vi "LinearKFLOP.vi"(8 "Array":dbl[](array[numeric]), 10 "error in (no error)":errorcluster, 11 "new reference":refnum<k24>) -> (2 "error out":errorcluster, 3 "new reference 2":refnum<k24>)   [LabVIEW 2017]
uses:
  C:/KMotion434/KMotion/Release/KMotion_dotNet.dll
panel:
  in  "y":bool
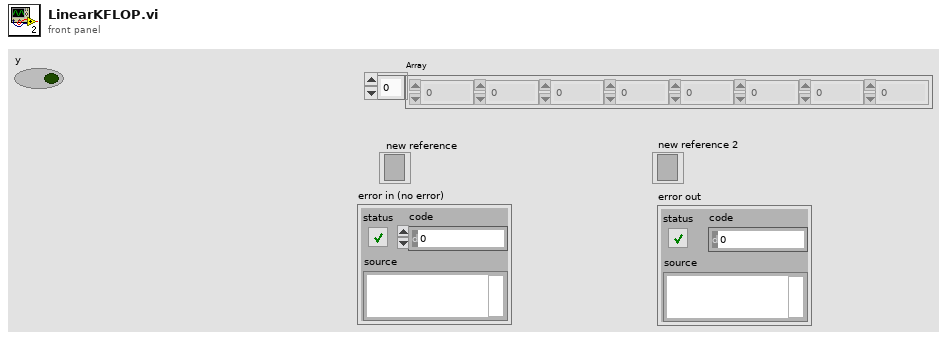
[diagram p1: front panel]
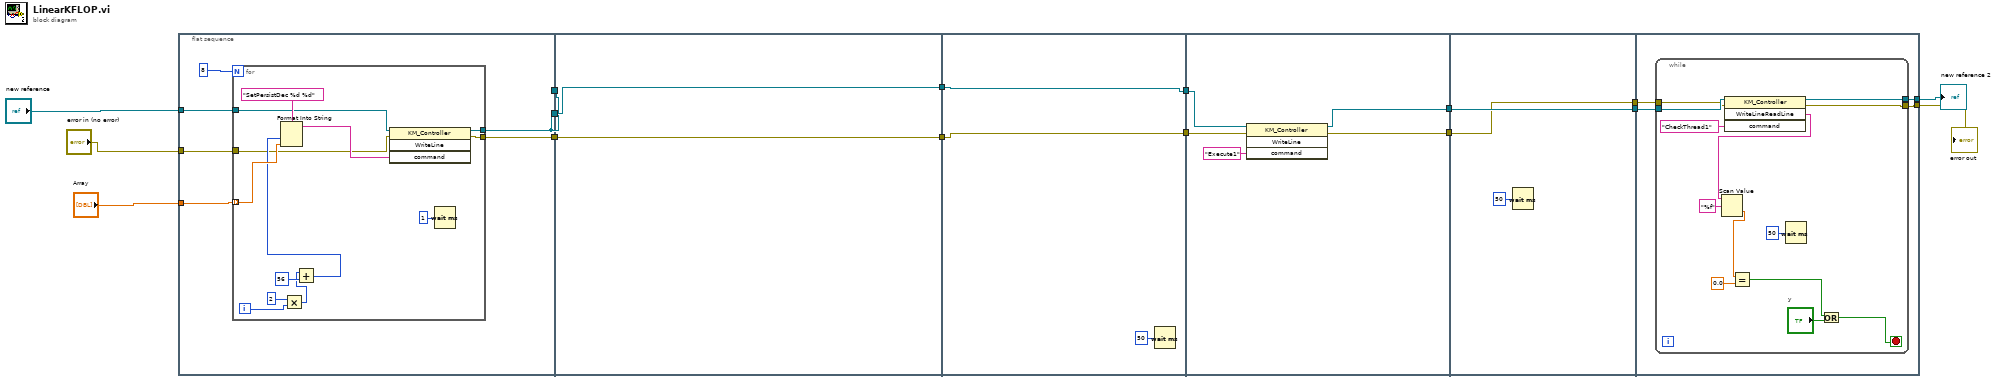
[diagram p0: block diagram]
diagram:
  n1 = flat-sequence {
    tunnel: "new reference" -> [w21]
    tunnel: "Array" -> [w20]
    tunnel: [w19] -> w15
    tunnel: [w19] -> w14
    tunnel: "error in (no error)" -> [w18]
    tunnel: [w17] -> w7
    tunnel: w15 -> [_]
    tunnel: w14 -> [w37]
    tunnel: [w37] -> w13
    tunnel: [w36] -> w8
    tunnel: w7 -> [w36]
    tunnel: [w39] -> w16
    tunnel: w13 -> [w39]
    tunnel: w8 -> [w38]
    tunnel: [w38] -> w6
    tunnel: w16 -> [w45]
    tunnel: [w44] -> w12
    tunnel: w6 -> [w41]
    tunnel: [w42] -> w4
    tunnel: w12 -> [w48]
    tunnel: [w48] -> w11
    tunnel: [w46] -> w5
    tunnel: w4 -> [w46]
    tunnel: w11 -> [w52]
    tunnel: w5 -> [w51]
    tunnel: [w50] -> w3
    tunnel: [w49] -> w2
    frame #0 {
      n2 = for {
        N: 8 -> [_]
        tunnel: w21 -> [w29]
        tunnel: w20 -> [w33] mode=indexing
        tunnel: [w32] -> w19
        tunnel: w18 -> [w24]
        tunnel: [w23] -> w17
        i -> [w27]
        n3 = Multiply(x=2, y=w27) -> (x*y=w26:i32)
        n4 = Add(x=w26, y=56) -> (x+y=w30:i32)
        n5 = Format Into String(format string="SetPersistDec %d %d" ("command"), w30, w33) -> (resulting string=w35:string)  [unwired: 2 in, 1 out]
        n6 = invoke class="KM_Controller" method="WriteLine"(reference=w29, error in=w24, "command"=w35) -> (reference out=w32:refnum<k24>, error out=w23:errorcluster)  [unwired: 1 in, 2 out]
        n7 = Wait (ms)(milliseconds to wait=u32 1) -> ()  [unwired: 1 out]
      }
    }
    frame #1 {
    }
    frame #2 {
      n8 = Wait (ms)(milliseconds to wait=u32 50) -> ()  [unwired: 1 out]
    }
    frame #3 {
      n9 = invoke class="KM_Controller" method="WriteLine"(reference=w45, error in=w41, "command"="Execute1") -> (reference out=w44:refnum<k24>, error out=w42:errorcluster)  [unwired: 1 in, 2 out]
    }
    frame #4 {
      n10 = Wait (ms)(milliseconds to wait=u32 50) -> ()  [unwired: 1 out]
    }
    frame #5 {
      n11 = while {
        tunnel: w52 -> [w65]
        tunnel: w51 -> [w55]
        tunnel: [w54] -> w50
        tunnel: [w53] -> w49
        stop <- w60 stop-if-true
        n12 = invoke class="KM_Controller" method="WriteLineReadLine"(reference=w65, error in=w55, "command"="CheckThread1") -> (reference out=w54:refnum<k24>, error out=w53:errorcluster, "WriteLineReadLine"=w61:string)  [unwired: 1 in, 1 out]
        n13 = Scan Value(string=w61, format string="%f") -> (value=w57:dbl)  [unwired: 1 in, 1 out]
        n14 = Equal?(x=w57, y=0.0) -> (x = y?=w59:bool)
        n15 = Wait (ms)(milliseconds to wait=u32 50) -> ()  [unwired: 1 out]
        n16 = Or(x=w59, y="y") -> (x .or. y?=w60:bool)
      }
    }
  }
  "new reference 2" <- w3
  "error out" <- w2
